vi "s_TurnTrapsOnOffWithJoystick.vi"(8 "Error In":errorcluster, 9 "Shutter Control Reference Cluster":T1, 10 "NewJoystButtInfo":T2, 11 "OldJoystButtInfo":T2) -> (0 "Error Out":errorcluster)   [LabVIEW 2012]
uses:
  <vilib>/DAQmx/create/channels.llb/DAQmx Create Channel (DO-Digital Output).vi
  <vilib>/DAQmx/read.llb/DAQmx Read (Digital Bool 1Line 1Point).vi
  <vilib>/DAQmx/write.llb/DAQmx Write (Digital Bool 1Line 1Point).vi
panel:
  # "Button 4 for Trap A\nButton 5 for Trap B"
  # "Whenever the B4 or B5 are pressed, open/close shutter to turn on/off \nthe respective optical trap"
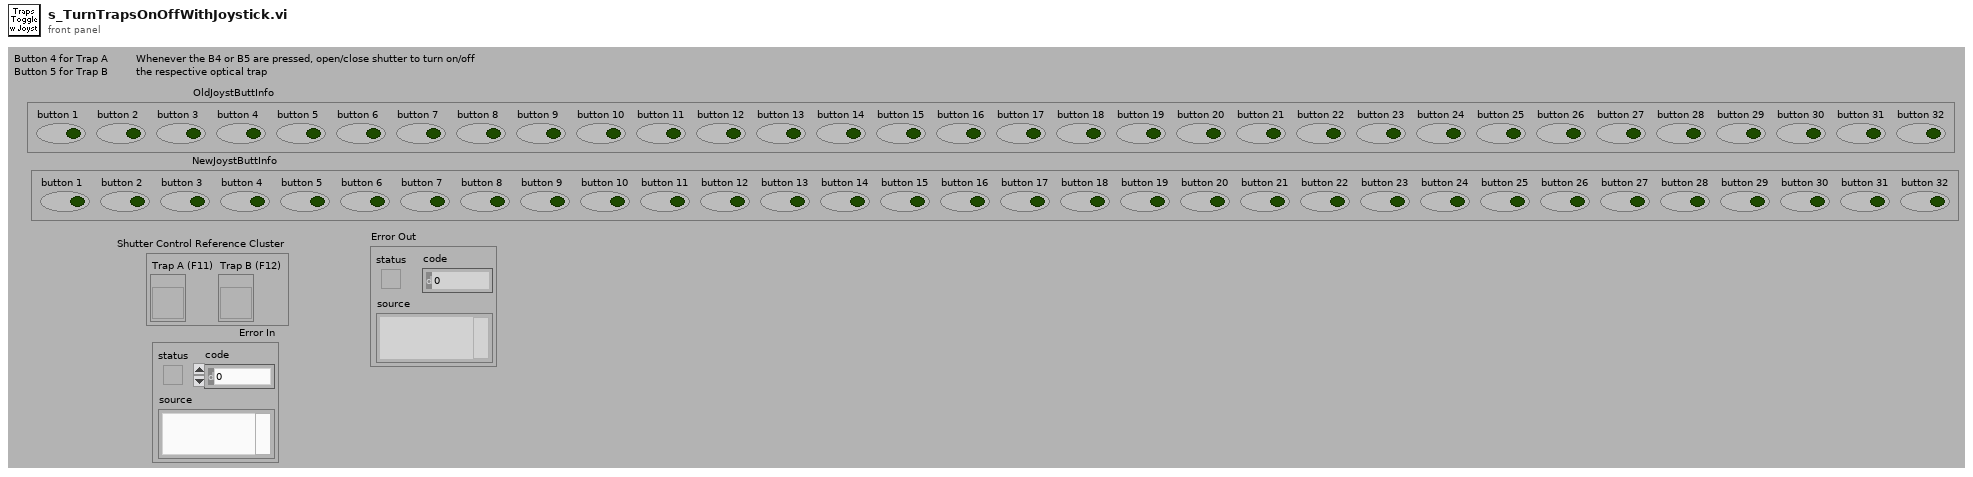
[diagram p1: front panel]
types:
  T1 = cluster{"Trap A (F11)":refnum<vi>, "Trap B (F12)":refnum<vi>}
  T2 = cluster{"button 1":bool, "button 2":bool, "button 3":bool, "button 4":bool, "button 5":bool, "button 6":bool, "button 7":bool, "button 8":bool, "button 9":bool, "button 10":bool, "button 11":bool, "button 12":bool, "button 13":bool, "button 14":bool, "button 15":bool, "button 16":bool, "button 17":bool, "button 18":bool, "button 19":bool, "button 20":bool, "button 21":bool, "button 22":bool, "button 23":bool, "button 24":bool, "button 25":bool, "button 26":bool, "button 27":bool, "button 28":bool, "button 29":bool, "button 30":bool, "button 31":bool, "button 32":bool}
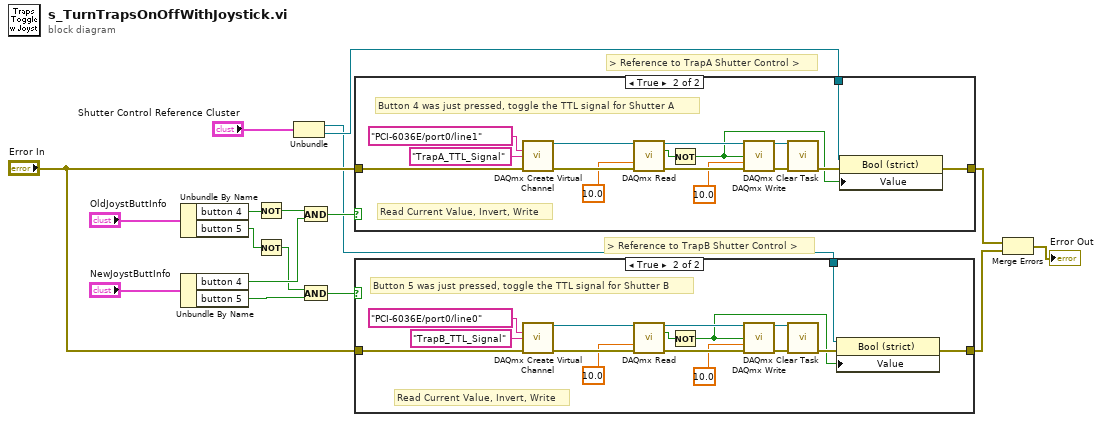
[diagram p0: block diagram]
diagram:
  # "> Reference to TrapB Shutter Control >"
  # "> Reference to TrapA Shutter Control >"
  n1 = Unbundle By Name("OldJoystButtInfo") -> ("button 4"=w15:bool, "button 5"=w11:bool)
  n2 = Unbundle By Name("NewJoystButtInfo") -> ("button 4"=w14:bool, "button 5"=w10:bool)
  n3 = Not(x=w15) -> (.not. x?=w13:bool)
  n4 = Not(x=w11) -> (.not. x?=w9:bool)
  n5 = Unbundle("Shutter Control Reference Cluster") -> ("Trap A (F11)"=w1:refnum<vi>, "Trap B (F12)"=w2:refnum<vi>)
  n6 = And(x=w13, y=w14) -> (x .and. y?=w12:bool)
  n7 = And(x=w9, y=w10) -> (x .and. y?=w8:bool)
  n8 = case shown="True" w12 {
    tunnel: [w18 w21] -> w4
    tunnel: "Error In" -> [w18 w23]
    tunnel: w2 -> [_ w19]
    frame False {
    }
    frame True {
      # "Read Current Value, Invert, Write"
      # "Button 4 was just pressed, toggle the TTL signal for Shutter A"
      n9 = call-poly <vilib>:"DAQmx Create Virtual Channel.vi"("lines"=tag "PCI-6036E/port0/line1", "name to assign"="TrapA_TTL_Signal", "error in"=w23) -> ("task out"=w29:refnum<k21>, "error out"=w33:errorcluster)  [unwired: 11 in]
      n10 = call-poly <vilib>:"DAQmx Read.vi"("task/channels in"=w29, "timeout"=10.0, "error in"=w33) -> ("task out"=w31:refnum<k21>, "data"=w30:bool, "error out"=w34:errorcluster)  [unwired: 10 in]
      n11 = Not(x=w30) -> (.not. x?=w20:bool)
      n12 = call-poly <vilib>:"DAQmx Write.vi"("task/channels in"=w31, "data"=w20, "timeout"=10.0, "error in"=w34) -> ("task out"=w27:refnum<k21>, "error out"=w28:errorcluster)  [unwired: 9 in, 1 out]
      n13 = call <vilib>:"DAQmx Clear Task.vi"("task in"=w27, "error in"=w28) -> ("error out"=w22:errorcluster)  [unwired: 13 in]
      n14 = property class="Bool (strict)"(reference=w19, error in=w22, "Value"=w20) -> (error out=w21:errorcluster)  [unwired: 1 out]
    }
  }
  n15 = case shown="True" w8 {
    tunnel: [w35 w38] -> w3
    tunnel: "Error In" -> [w35 w40]
    tunnel: w1 -> [_ w36]
    frame False {
    }
    frame True {
      # "Read Current Value, Invert, Write"
      # "Button 5 was just pressed, toggle the TTL signal for Shutter B"
      n16 = call-poly <vilib>:"DAQmx Create Virtual Channel.vi"("lines"=tag "PCI-6036E/port0/line0", "name to assign"="TrapB_TTL_Signal", "error in"=w40) -> ("task out"=w46:refnum<k21>, "error out"=w50:errorcluster)  [unwired: 11 in]
      n17 = call-poly <vilib>:"DAQmx Read.vi"("task/channels in"=w46, "timeout"=10.0, "error in"=w50) -> ("task out"=w48:refnum<k21>, "data"=w47:bool, "error out"=w51:errorcluster)  [unwired: 10 in]
      n18 = Not(x=w47) -> (.not. x?=w37:bool)
      n19 = call-poly <vilib>:"DAQmx Write.vi"("task/channels in"=w48, "data"=w37, "timeout"=10.0, "error in"=w51) -> ("task out"=w44:refnum<k21>, "error out"=w45:errorcluster)  [unwired: 9 in, 1 out]
      n20 = call <vilib>:"DAQmx Clear Task.vi"("task in"=w44, "error in"=w45) -> ("error out"=w39:errorcluster)  [unwired: 13 in]
      n21 = property class="Bool (strict)"(reference=w36, error in=w39, "Value"=w37) -> (error out=w38:errorcluster)  [unwired: 1 out]
    }
  }
  n22 = Merge Errors(w4, w3) -> (→"Error Out":errorcluster)
